vi "create configuration.vi"(8 "error in":errorcluster, 11 "lvlibretls configurable context in":refnum<class "lvlibretls configurable context.lvclass">) -> (0 "error out":errorcluster, 3 "lvlibretls configurable context out":refnum<class "lvlibretls configurable context.lvclass">)   [LabVIEW 2016, in "lvlibretls configurable context.lvclass"]
uses:
  lvlibretls configurable context.lvclass
  lvlibretls configurable context.lvclass/lvlibretls configurable context.ctl
  lv tls dll.lvlib
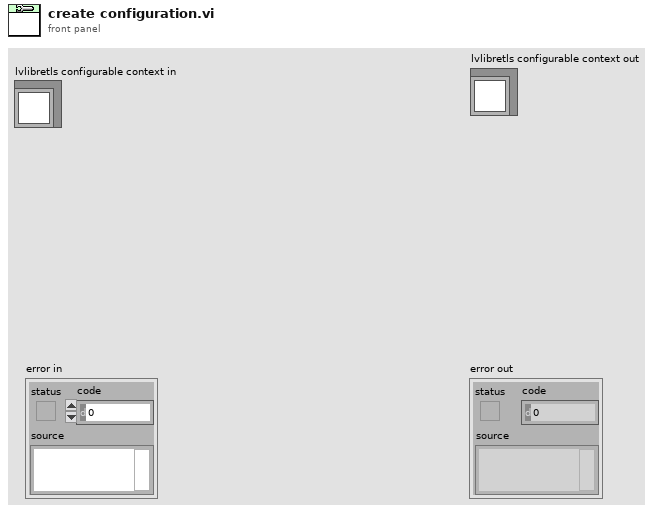
[diagram p1: front panel]
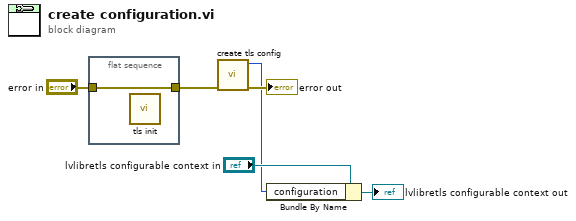
[diagram p0: block diagram]
diagram:
  n1 = flat-sequence {
    tunnel: "error in" -> [w7]
    tunnel: [w7] -> w1
    frame #0 {
      n2 = call "tls init.vi"() -> ()  [unwired: 11 in, 1 out]
    }
  }
  n3 = call "create tls config.vi"("error in"=w1) -> ("error out"=→"error out":errorcluster, "config out"=w3:u64)  [unwired: 9 in]
  n4 = Bundle By Name(cluster="lvlibretls configurable context in", "configuration"=w3) -> (→"lvlibretls configurable context out":refnum<class "lvlibretls configurable context.lvclass">)
